vi "Get Video Image.vi"(8 "error in (no error)":errorcluster, 9 "Wait For Next Image?":bool=TRUE, 11 "Reference In":T1) -> (0 "error out":errorcluster, 1 "Video Image Pixels (U32)":u32[][](array[numeric]), 2 "Video Image":T2(plugin-control), 3 "Reference Out":T1)   [LabVIEW 2010]
uses:
  <vilib>/vision/Image Controls.llb/IMAQ Image.ctl
  Microsoft.Research.Kinect
panel:
  out "Image Is New?":bool
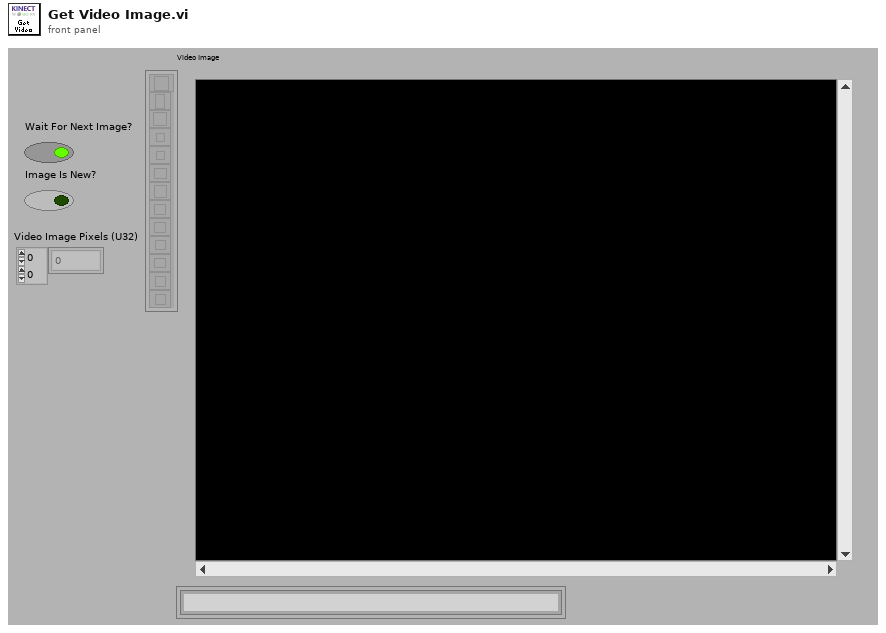
[diagram p1: front panel]
types:
  T1 = cluster{cluster{"queue out":refnum<queue>, "queue out":refnum<queue>}, cluster{"new reference":refnum<k24>, "DepthStream":refnum<k24>, "VideoStream":refnum<k24>, "Event Callback":refnum<k27>, "Event Callback":refnum<k27>}}
  T2 = typedef "IMAQ Image.ctl" = refnum<image>
  T3 = cluster{"queue out":refnum<queue>, "queue out":refnum<queue>}
  T4 = typedef "Image Type" = u32
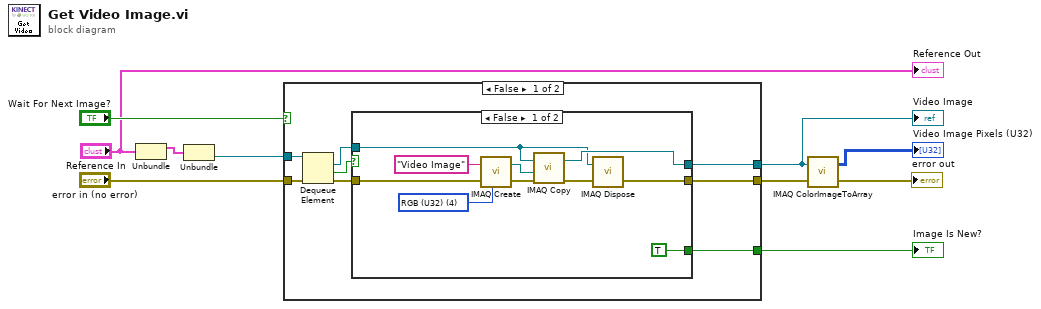
[diagram p0: block diagram]
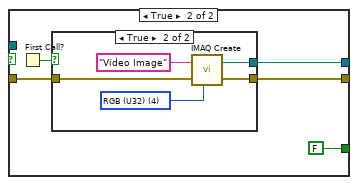
[diagram p2: hidden frame]
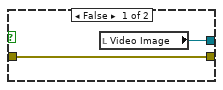
[diagram p3: hidden frame]
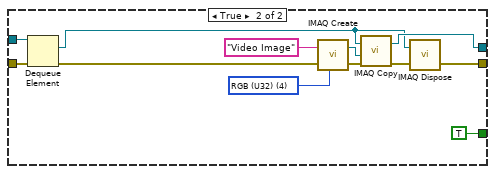
[diagram p4: hidden frame]
diagram:
  n1 = Unbundle("Reference In") -> (w1:T3)  [unwired: 1 out]
  n2 = Unbundle(w1) -> ("queue out"=w2:refnum<queue>)  [unwired: 1 out]
  n3 = case shown="False" "Wait For Next Image?" {
    tunnel: "error in (no error)" -> [w14 w52]
    tunnel: [w16 w46] -> w4
    tunnel: [w17 w42] -> w5
    tunnel: [w18 TRUE] -> w7
    tunnel: w2 -> [w15 w50]
    frame False {
      n4 = Dequeue Element(queue=w15, error in (no error)=w14) -> (element=w11:T2, timed out?=w12:bool, error out=w13:errorcluster)  [unwired: 1 in, 1 out]
      n5 = case shown="False" w12 {
        tunnel: [w22 w29] -> w16
        tunnel: w13 -> [w19 w31]
        tunnel: [w21 w30] -> w17
        tunnel: [TRUE FALSE] -> w18
        tunnel: w11 -> [w20 _]
        frame False {
          w24 = T4 4 items=["Grayscale (U8)", "Grayscale (I16)", "Grayscale (SGL)", "Complex (CSG)", "RGB (U32)", "HSL (U32)", "RGB (U64)", "Grayscale (U16)"] ("Image Type")
          n6 = call "IMAQ Create"("Image Name"="Video Image", "Image Type"=w24, "error in (no error)"=w19) -> ("New Image"=w26:T2, "error out"=w25:errorcluster)  [unwired: 2 in]
          n7 = call "IMAQ Copy"("error in (no error)"=w25, "Image Dst"=w26, "Image Src"=w20) -> ("error out"=w23:errorcluster, "Image Dst Out"=w22:T2)  [unwired: 3 in]
          n8 = call "IMAQ Dispose"("Image"=w20, "error in (no error)"=w23) -> ("error out"=w21:errorcluster)  [unwired: 4 in]
        }
        frame True {
          n9 = First Call?() -> (First Call?: T/F=w32:bool)
          n10 = case shown="True" w32 {
            tunnel: [w35 w36] -> w29
            tunnel: w31 -> [w34 w38]
            tunnel: [w34 w37] -> w30
            frame False {
              n11 = local read "Video Image"() -> (w35:T2)
            }
            frame True {
              w39 = T4 4 items=["Grayscale (U8)", "Grayscale (I16)", "Grayscale (SGL)", "Complex (CSG)", "RGB (U32)", "HSL (U32)", "RGB (U64)", "Grayscale (U16)"] ("Image Type")
              n12 = call "IMAQ Create"("Image Name"="Video Image", "Image Type"=w39, "error in (no error)"=w38) -> ("New Image"=w36:T2, "error out"=w37:errorcluster)  [unwired: 2 in]
            }
          }
        }
      }
    }
    frame True {
      w44 = T4 4 items=["Grayscale (U8)", "Grayscale (I16)", "Grayscale (SGL)", "Complex (CSG)", "RGB (U32)", "HSL (U32)", "RGB (U64)", "Grayscale (U16)"] ("Image Type")
      n13 = Dequeue Element(queue=w50, error in (no error)=w52) -> (element=w41:T2, error out=w48:errorcluster)  [unwired: 1 in, 2 out]
      n14 = call "IMAQ Create"("Image Name"="Video Image", "Image Type"=w44, "error in (no error)"=w48) -> ("New Image"=w47:T2, "error out"=w45:errorcluster)  [unwired: 2 in]
      n15 = call "IMAQ Copy"("error in (no error)"=w45, "Image Dst"=w47, "Image Src"=w41) -> ("error out"=w43:errorcluster, "Image Dst Out"=w46:T2)  [unwired: 3 in]
      n16 = call "IMAQ Dispose"("Image"=w41, "error in (no error)"=w43) -> ("error out"=w42:errorcluster)  [unwired: 4 in]
    }
  }
  "Video Image" <- w4
  "Image Is New?" <- w7
  n17 = call "IMAQ ColorImageToArray"("Image"=w4, "error in (no error)"=w5) -> ("Image Pixels (U32)"=→"Video Image Pixels (U32)":u32[][], "error out"=→"error out":errorcluster)  [unwired: 2 in, 1 out]
  "Reference Out" <- "Reference In"
